vi "Compute Angle (SubVI).vi"(8 "N Points":u16, 11 "Start":bool) -> (1 "Angle Valid?":bool, 2 "Angle":fxp<+/-,16,3> format="%.14g", 3 "Done?":bool)   [LabVIEW 2015]
uses:
  Controls (FPGA)/Compute Angle.ctl
  <vilib>/rvi/FXPMathLib/FxpAtan2/subVIs/nifxpmath_Atan2_SimConfig.ctl
  <vilib>/rvi/Emulation/niFpgaProcessEmulError.vi
  <vilib>/rvi/Memory/Memory_Emulation/nirvimemoryFastEmulation.vi
  <vilib>/rvi/Memory/Memory_Emulation/nirvimemoryEmulation.vi
  <vilib>/rvi/Emulation/niFpgaEmulationIsFPGAContextNoSignature.vi
  <vilib>/rvi/DataTransferAndStorage/Container/Common/niFpgaContainerGetUniqueNameForEmu.vi
  <vilib>/rvi/Emulation/niFpgaSctlEmulationGetInTimedLoop.vi
  <vilib>/rvi/errors/nirviReportUnexpectedCaseInternalError (U32).vi
  <vilib>/rvi/FXPMathLib/FxpAtan2/simVIs/DllFxpAtan2Temp_sub.vi
  <vilib>/rvi/DataTransferAndStorage/Container/XNode/niFpgaContainer.xnode
  <vilib>/rvi/FXPMathLib/FxpAtan2/XNode/nifxpmath_Atan2.xnode
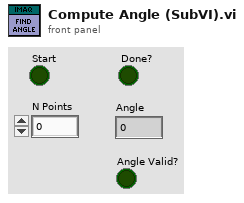
[diagram p1: front panel]
types:
  T1 = typedef "Compute Angle.ctl" = enum16{"Wait", "Read Contour Points"}
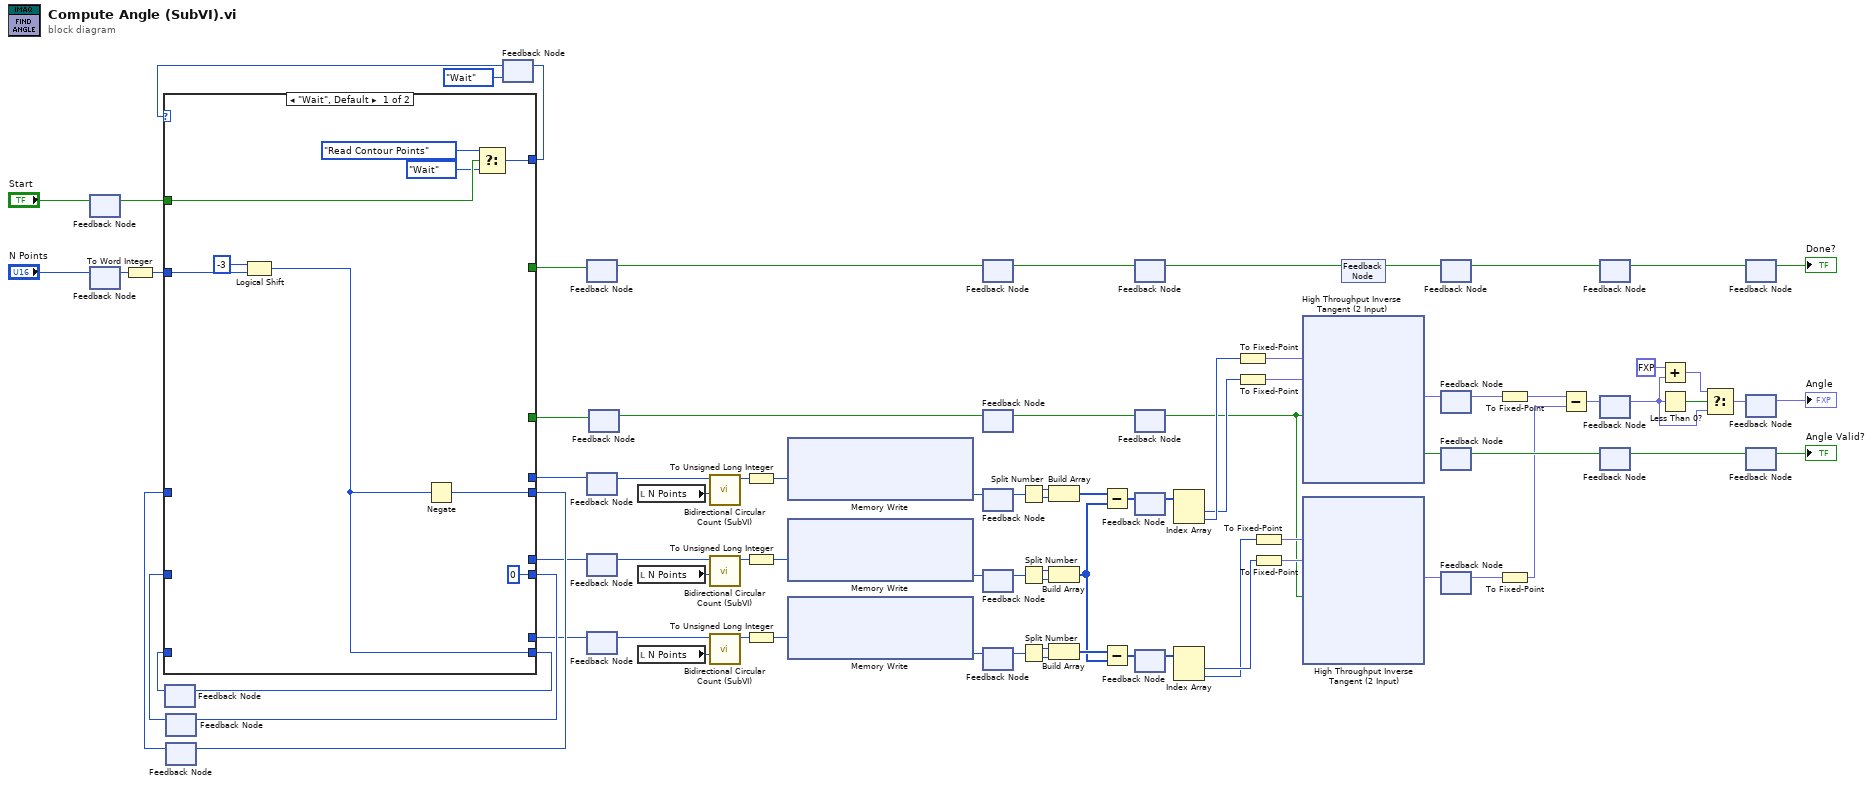
[diagram p0: block diagram]
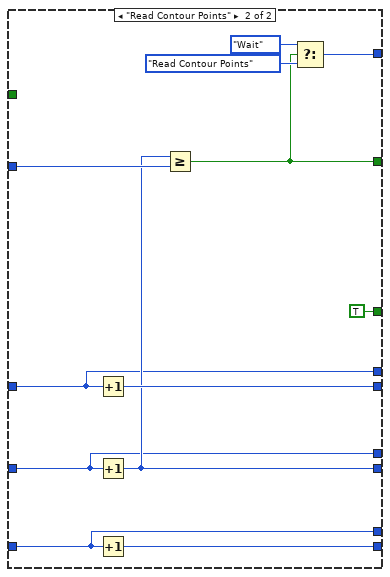
[diagram p2: hidden frame]
diagram:
  n1 = feedback-in #1("Start") -> ()
  n2 = feedback #1() -> (w72:bool)  [unwired: 1 in]
  n3 = feedback-in #2("N Points") -> ()
  n4 = feedback #2() -> (w69:u16)  [unwired: 1 in]
  n5 = To Word Integer(number=w69) -> (16bit integer=w68:i16)
  n6 = feedback #3() -> (w67:i16)  [unwired: 1 in]
  n7 = feedback #4() -> (w77:i16)  [unwired: 1 in]
  n8 = feedback #5() -> (w76:i16)  [unwired: 1 in]
  n9 = feedback #6(Compute_Angle."Wait") -> (w75:T1)
  n10 = case shown="\"Wait\", Default" w75 {
    tunnel: [w94 w106] -> w74
    tunnel: w76 -> [_ w95]
    tunnel: [w86 w105] -> w80
    tunnel: [i16 0 ("Count Out") w102] -> w79
    tunnel: w77 -> [_ w96]
    tunnel: [_ w99] -> w78
    tunnel: w72 -> [w93 _]
    tunnel: w68 -> [w89 w104]
    tunnel: [w87 w103] -> w66
    tunnel: w67 -> [_ w97]
    tunnel: [_ TRUE] -> w56
    tunnel: [_ w97] -> w3
    tunnel: [_ w96] -> w2
    tunnel: [_ w95] -> w1
    frame "Wait", Default {
      n11 = Logical Shift(y=i16 -3, x=w89) -> (x << y=w87:i16)
      n12 = Negate(x=w87) -> (-x=w86:i16)
      n13 = Select(t=Compute_Angle."Read Contour Points", s=w93, f=Compute_Angle."Wait") -> (s? t:f=w94:T1)
    }
    frame "Read Contour Points" {
      n14 = Increment(x=w95) -> (x+1=w105:i16)
      n15 = Increment(x=w96) -> (x+1=w102:i16)
      n16 = Increment(x=w97) -> (x+1=w103:i16)
      n17 = Greater Or Equal?(x=w102, y=w104) -> (x >= y?=w99:bool)
      n18 = Select(t=Compute_Angle."Wait", s=w99, f=Compute_Angle."Read Contour Points") -> (s? t:f=w106:T1)
    }
  }
  n19 = feedback-in #3(w66) -> ()
  n20 = feedback-in #4(w79) -> ()
  n21 = feedback-in #5(w80) -> ()
  n22 = feedback-in #6(w74) -> ()
  n23 = feedback #7() -> (w83:bool)  [unwired: 1 in]
  n24 = feedback-in #7(w78) -> ()
  n25 = feedback-in #8(w1) -> ()
  n26 = feedback #8() -> (w62:i16)  [unwired: 1 in]
  n27 = feedback-in #9(w2) -> ()
  n28 = feedback #9() -> (w61:i16)  [unwired: 1 in]
  n29 = feedback-in #10(w3) -> ()
  n30 = feedback #10() -> (w60:i16)  [unwired: 1 in]
  n31 = feedback #11() -> (w40:bool)  [unwired: 1 in]
  n32 = feedback-in #11(w56) -> ()
  n33 = local read "N Points"() -> (w59:u16)
  n34 = local read "N Points"() -> (w58:u16)
  n35 = local read "N Points"() -> (w57:u16)
  n36 = call "Bidirectional Circular Count (SubVI).vi"("Max. Count"=w59, "Count In"=w62) -> ("Count Out"=w65:i16)  [unwired: 9 in]
  n37 = call "Bidirectional Circular Count (SubVI).vi"("Max. Count"=w58, "Count In"=w61) -> ("Count Out"=w64:i16)  [unwired: 9 in]
  n38 = call "Bidirectional Circular Count (SubVI).vi"("Max. Count"=w57, "Count In"=w60) -> ("Count Out"=w63:i16)  [unwired: 9 in]
  n39 = To Unsigned Long Integer(number=w65) -> (unsigned 32bit integer=w81:u32)
  n40 = To Unsigned Long Integer(number=w64) -> (unsigned 32bit integer=w82:u32)
  n41 = To Unsigned Long Integer(number=w63) -> (unsigned 32bit integer=w71:u32)
  n42 = xnode ("Memory Write")("Address"=w81) -> ("Data"=w55:u32)  [unwired: 1 in, 1 out]
  n43 = xnode ("Memory Write")("Address"=w82) -> ("Data"=w54:u32)  [unwired: 1 in, 1 out]
  n44 = xnode ("Memory Write")("Address"=w71) -> ("Data"=w53:u32)  [unwired: 1 in, 1 out]
  n45 = feedback-in #12(w83) -> ()
  n46 = feedback #12() -> (w20:bool)  [unwired: 1 in]
  n47 = feedback-in #13(w40) -> ()
  n48 = feedback #13() -> (w29:bool)  [unwired: 1 in]
  n49 = feedback-in #14(w55) -> ()
  n50 = feedback #14() -> (w46:u32)  [unwired: 1 in]
  n51 = feedback-in #15(w54) -> ()
  n52 = feedback #15() -> (w45:u32)  [unwired: 1 in]
  n53 = feedback-in #16(w53) -> ()
  n54 = feedback #16() -> (w44:u32)  [unwired: 1 in]
  n55 = Split Number(x=w46) -> (hi(x)=w52:u16, lo(x)=w51:u16)
  n56 = Split Number(x=w45) -> (hi(x)=w50:u16, lo(x)=w49:u16)
  n57 = Split Number(x=w44) -> (hi(x)=w48:u16, lo(x)=w47:u16)
  n58 = Build Array(w52, w51) -> (w43:u16[])
  n59 = Build Array(w50, w49) -> (w41:u16[])
  n60 = Build Array(w48, w47) -> (w42:u16[])
  n61 = Subtract(x=w43, y=w41) -> (x-y=w39:u16[])
  n62 = Subtract(x=w42, y=w41) -> (x-y=w30:u16[])
  n63 = feedback-in #17(w20) -> ()
  n64 = feedback #17() -> (w21:bool)  [unwired: 1 in]
  n65 = feedback-in #18(w29) -> ()
  n66 = feedback #18() -> (w26:bool)  [unwired: 1 in]
  n67 = feedback-in #19(w39) -> ()
  n68 = feedback #19() -> (w28:u16[])  [unwired: 1 in]
  n69 = feedback-in #20(w30) -> ()
  n70 = feedback #20() -> (w27:u16[])  [unwired: 1 in]
  n71 = Index Array(array=w28) -> (element #1=w35:u16, element #2=w37:u16)  [unwired: 2 in]
  n72 = Index Array(array=w27) -> (element #1=w34:u16, element #2=w32:u16)  [unwired: 2 in]
  n73 = To Fixed-Point(number=w37) -> (fixed-point=w38:fxp<+/-,16,16>)  [unwired: 1 in]
  n74 = To Fixed-Point(number=w35) -> (fixed-point=w36:fxp<+/-,16,16>)  [unwired: 1 in]
  n75 = To Fixed-Point(number=w32) -> (fixed-point=w31:fxp<+/-,16,16>)  [unwired: 1 in]
  n76 = To Fixed-Point(number=w34) -> (fixed-point=w33:fxp<+/-,16,16>)  [unwired: 1 in]
  n77 = xnode "High Throughput Inverse Tangent (2 Input)"("y"=w38, "x"=w36, "input valid"=w26) -> ("atan2(y,x) (pi)"=w25:fxp<+/-,16,2>, "output valid"=w7:bool)  [unwired: 1 in, 1 out]
  n78 = xnode "High Throughput Inverse Tangent (2 Input)"("y"=w31, "x"=w33, "input valid"=w26) -> ("atan2(y,x) (pi)"=w24:fxp<+/-,16,2>)  [unwired: 1 in, 2 out]
  n79 = feedback-in #21(w21) -> ()
  n80 = feedback #21() -> (w19:bool)  [unwired: 1 in]
  n81 = feedback-in #22(w19) -> ()
  n82 = feedback #22() -> (w18:bool)  [unwired: 1 in]
  n83 = feedback-in #23(w25) -> ()
  n84 = feedback #23() -> (w23:fxp<+/-,16,2>)  [unwired: 1 in]
  n85 = feedback #24() -> (w85:bool)  [unwired: 1 in]
  n86 = feedback-in #24(w7) -> ()
  n87 = feedback-in #25(w24) -> ()
  n88 = feedback #25() -> (w22:fxp<+/-,16,2>)  [unwired: 1 in]
  n89 = To Fixed-Point(number=w23) -> (fixed-point=w9:fxp<+/-,16,3>)  [unwired: 1 in]
  n90 = To Fixed-Point(number=w22) -> (fixed-point=w8:fxp<+/-,16,3>)  [unwired: 1 in]
  n91 = Subtract(x=w9, y=w8) -> (x-y=w15:fxp<+/-,16,3>)
  n92 = feedback-in #26(w18) -> ()
  n93 = feedback #26() -> (w13:bool)  [unwired: 1 in]
  n94 = feedback-in #27(w15) -> ()
  n95 = feedback #27() -> (w12:fxp<+/-,16,3>)  [unwired: 1 in]
  n96 = feedback-in #28(w85) -> ()
  n97 = feedback #28() -> (w11:bool)  [unwired: 1 in]
  n98 = Add(x=fxp<+/-,16,3> 2.0, y=w12) -> (x+y=w16:fxp<+/-,16,3>)
  n99 = Less Than 0?(x=w12) -> (x < 0?=w17:bool)
  n100 = Select(t=w16, s=w17, f=w12) -> (s? t:f=w10:fxp<+/-,16,3>)
  n101 = feedback-in #29(w13) -> ()
  n102 = feedback #29() -> (→"Done?":bool)  [unwired: 1 in]
  n103 = feedback-in #30(w10) -> ()
  n104 = feedback #30() -> (→"Angle":fxp<+/-,16,3>)  [unwired: 1 in]
  n105 = feedback-in #31(w11) -> ()
  n106 = feedback #31() -> (→"Angle Valid?":bool)  [unwired: 1 in]
